vi "Read TrayStatus.vi"(8 "error in (no error)":errorcluster, 10 "F1/T2":bool, 11 "LaserDetect01 in":refnum<class "LaserDetect01.lvclass">) -> (0 "error out":errorcluster, 1 "Arr_TrayST":bool[][](array[boolean]), 2 "Arr_Tray":cluster{"X":sgl, "Y":sgl}[][](array[cluster]), 3 "LaserDetect01 out":refnum<class "LaserDetect01.lvclass">)   [LabVIEW 2019, in "LaserDetect01.lvclass"]
uses:
  LaserDetect01.lvclass
  FlowIOCtrl.lvclass
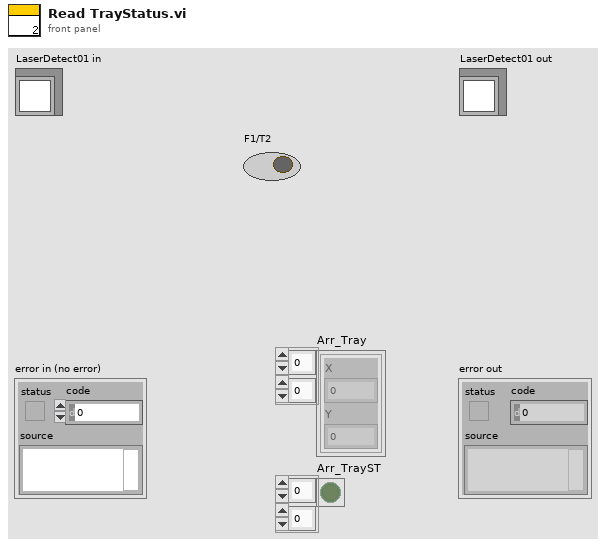
[diagram p1: front panel]
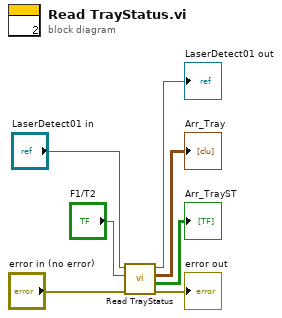
[diagram p0: block diagram]
diagram:
  n1 = call-parent "Read TrayStatus.vi"("error in (no error)"="error in (no error)", "F1/T2"="F1/T2", "Station Action in"="LaserDetect01 in") -> ("error out"=→"error out":errorcluster, "Arr_TrayST"=→"Arr_TrayST":bool[][], "Arr_Tray"=→"Arr_Tray":cluster{"X":sgl, "Y":sgl}[][], "Station Action out"=→"LaserDetect01 out":refnum<class "LaserDetect01.lvclass">)  [unwired: 5 in]
